vi "CB Get Range.vi"(4 "CB type":u16, 6 "CB size":i32, 9 "i":i32, 10 "Write Targets (1b)":dbl[][](array[numeric]), 11 "Write Targets (multi-bit)":dbl[][](array[numeric])) -> (2 "Lower resistance (ohm)":dbl, 3 "Upper resistance (ohm)":dbl)   [LabVIEW 2018]
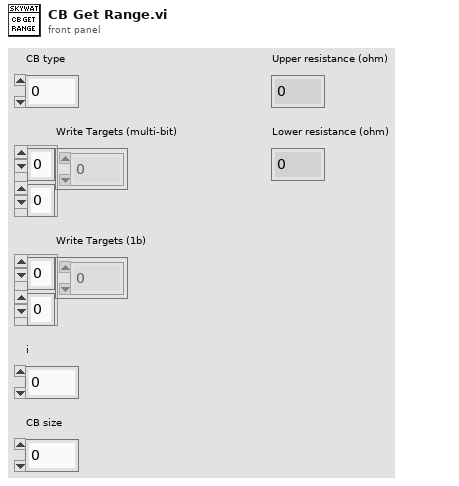
[diagram p1: front panel]
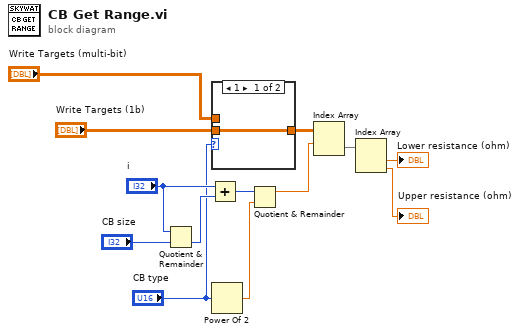
[diagram p0: block diagram]
diagram:
  n1 = Quotient & Remainder(x="i", y="CB size") -> (floor(x/y)=w10:i32)  [unwired: 1 out]
  n2 = Add(x="i", y=w10) -> (x+y=w7:i32)
  n3 = case shown="1" "CB type" {
    tunnel: "Write Targets (multi-bit)" -> [_ w15]
    tunnel: "Write Targets (1b)" -> [w14 _]
    tunnel: [w14 w15] -> w13
    frame 1 {
    }
    frame 2, Default {
    }
  }
  n4 = Power Of 2(x="CB type") -> (2^x=w1:dbl)
  n5 = Quotient & Remainder(x=w7, y=w1) -> (x-y*floor(x/y)=w3:dbl)  [unwired: 1 out]
  n6 = Index Array(array=w13, index (row)=w3) -> (element=w4:dbl[])  [unwired: 1 in]
  n7 = Index Array(array=w4) -> (element #1=→"Lower resistance (ohm)":dbl, element #2=→"Upper resistance (ohm)":dbl)  [unwired: 2 in]
